vi "merge_Count Up Down.vi"   [LabVIEW 2017, in "NI_FunctionBlockMergeVIs.lvlib"]
doc: "Reports the elapsed time, in milliseconds, since the first call or previous reset of the function block."
uses:
  <vilib>/functionblocks/NI_FunctionBlockMergeVIs.lvlib
  <vilib>/functionblocks/FB Core/FB Core.xnode
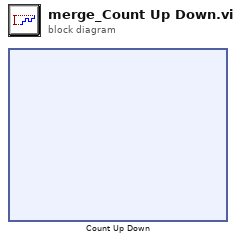
[diagram p0: block diagram]
diagram:
  n1 = xnode "Count Up Down"() -> ()  [unwired: 6 in, 4 out]
